vi "Configure Trigger (Timeout).vi"(0 "VISA resource name":refnum<visa-resource-name>, 1 "Timer (500E-12s)":dbl=5e-10, 5 "Source (0:Channel1)":u16(ring) items=["Channel1", "Channel2", "Channel3", "Channel4", "Digital Channel0", "Digital Channel1", "Digital Channel2", "Digital Channel3", "Digital Channel4", "Digital Channel5", "Digital Channel6", "Digital Channel7", "Digital Channel8", "Digital Channel9", "Digital Channel10", "Digital Channel11", "Digital Channel12", "Digital Channel13", "Digital Channel14", "Digital Channel15"], 7 "Trigger Level (0V)":dbl, 9 "Trigger Condition (0:Stays High)":u16(ring) items=["Stays High", "Stays Low", "Either"], 11 "error in (no error)":errorcluster, 12 "Trigger If Timeout (0:Occurs)":u16(ring) items=["Occurs", "Logic"], 13 "Trigger Event (0:A Event)":u16(ring) items=["A Event", "B Event"]) -> (4 "VISA resource name out":refnum<visa-resource-name>, 6 "Trigger Event Out":u16(ring) items=["A Event", "B Event"], 15 "error out":errorcluster)   [LabVIEW 2011, in "Tektronix 7000 Series.lvlib"]
doc: "Configures the timeout trigger settings for an oscilloscope. A timeout occurs when the pulse train stops in the selected state for longer than the specified time.\n\nTDS5000 ,TDS5000B,TDS6000 ,CSA7000 and TDS7000 series oscilloscopes don't support B Timeout Trigger."
uses:
  Tektronix 7000 Series.lvlib
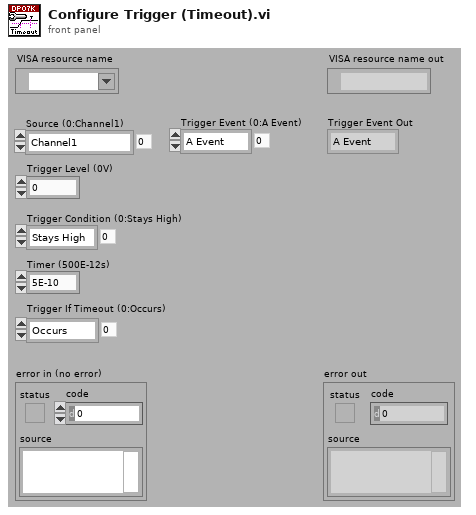
[diagram p1: front panel]
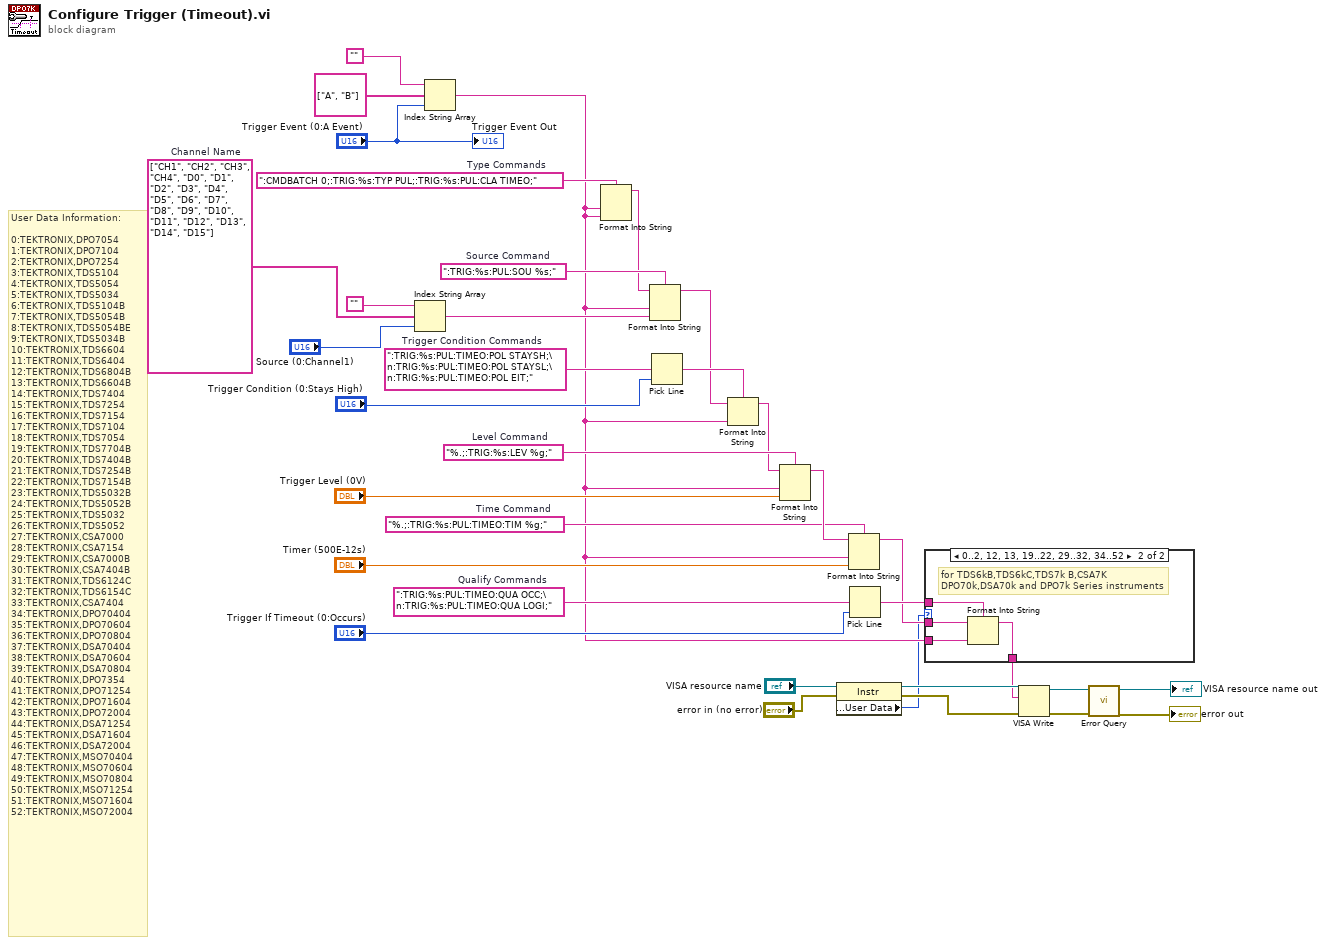
[diagram p0: block diagram]
diagram:
  w1 = string[] ["CH1", "CH2", "CH3", "CH4", "D0", "D1", "D2", "D3", "D4", "D5", "D6", "D7", "D8", "D9", "D10", "D11", "D12", "D13", "D14", "D15"]  # Channel Name
  w21 = "%.;:TRIG:%s:PUL:TIMEO:TIM %g;"  # Time Command
  w23 = "%.;:TRIG:%s:LEV %g;"  # Level Command
  w24 = ":TRIG:%s:PUL:TIMEO:QUA OCC;\n:TRIG:%s:PUL:TIMEO:QUA LOGI;"  # Qualify Commands
  w25 = ":TRIG:%s:PUL:TIMEO:POL STAYSH;\n:TRIG:%s:PUL:TIMEO:POL STAYSL;\n:TRIG:%s:PUL:TIMEO:POL EIT;"  # Trigger Condition Commands
  w26 = ":TRIG:%s:PUL:SOU %s;"  # Source Command
  w20 = ":CMDBATCH 0;:TRIG:%s:TYP PUL;:TRIG:%s:PUL:CLA TIMEO;"  # Type Commands
  # "User Data Information:\n\n0:TEKTRONIX,DPO7054\n1:TEKTRONIX,DPO7104\n2:TEKTRONIX,DPO7254\n3:TEKTRONIX,TDS5104\n4:TEKTRONIX,TDS5054\n5:TEKTRONIX,TDS5034\n6:TEKTRONIX,TDS5104B\n7:TEKTRONIX,TDS5054B\n8:TEKTRONIX,TDS5054BE\n9:TEKTRONIX,TDS5034B\n10:TEKTRONIX,TDS6604\n11:TEKTRONIX,TDS6404\n12:TEKTRONIX,TDS6804B\n13:TEKTRONIX,TDS6604B\n14:TEKTRONIX,TDS7404\n15:TEKTRONIX,TDS7254\n16:TEKTRONIX,TDS7154\n17:TEKTRONIX,TDS7104\n18:TEKTRONIX,TDS7054\n19:TEKTRONIX,TDS7704B\n20:TEKTRONIX,TDS7404B\n21:TEKTRONIX,TDS7254B\n22:TEKTRONIX,TDS7154B\n23:TEKTRONIX,TDS5032B\n24:TEKTRONIX,TDS5052B\n25:TEKTRONIX,TDS5032\n26:TEKTRONIX,TDS5052\n27:TEKTRONIX,CSA7000\n28:TEKTRONIX,CSA7154\n29:TEKTRONIX,CSA7000B\n30:TEKTRONIX,CSA7404B\n31:TEKTRONIX,TDS6124C\n32:TEKTRONIX,TDS6154C\n33:TEKTRONIX,CSA7404\n34:TEKTRONIX,DPO70404\n35:TEKTRONIX,DPO70604\n36:TEKTRONIX,DPO70804\n37:TEKTRONIX,DSA70404\n38:TEKTRONIX,DSA70604\n39:TEKTRONIX,DSA70804\n40:TEKTRONIX,DPO7354\n41:TEKTRONIX,DPO71254\n42:TEKTRONIX,DPO71604\n43:TEKTRONIX,DPO72004\n44:TEKTRONIX,DSA71254\n45:TEKTRONIX,DSA71604\n46:TEKTRONIX,DSA72004\n47:TEKTRONIX,MSO70404\n48:TEKTRONIX,MSO70604\n49:TEKTRONIX,MSO70804\n50:TEKTRONIX,MSO71254\n51:TEKTRONIX,MSO71604\n52:TEKTRONIX,MSO72004"
  n1 = Index String Array(1:"Source (0:Channel1)", 2:w1, 3:"") -> (0:w18:string)
  n2 = Index String Array(1:"Trigger Event (0:A Event)", 2:string[] ["A", "B"], 3:"" ("Empty String Constant")) -> (0:w10:string)
  n3 = Format Into String(format string=w20, w10, w10) -> (resulting string=w19:string)  [unwired: 2 in, 1 out]
  n4 = Format Into String(format string=w26, initial string=w19, w10, w18) -> (resulting string=w16:string)  [unwired: 1 in, 1 out]
  n5 = Pick Line(multi-line string=w25, line index="Trigger Condition (0:Stays High)") -> (output string=w17:string)  [unwired: 1 in]
  n6 = Format Into String(format string=w17, initial string=w16, w10) -> (resulting string=w15:string)  [unwired: 1 in, 1 out]
  n7 = Format Into String(format string=w23, initial string=w15, w10, "Trigger Level (0V)") -> (resulting string=w22:string)  [unwired: 1 in, 1 out]
  n8 = property class="Instr"(reference="VISA resource name", error in="error in (no error)") -> (reference out=w7:refnum<visa-resource-name>, error out=w6:errorcluster, "General Settings:User Data"=w5:u32)
  n9 = Format Into String(format string=w21, initial string=w22, w10, "Timer (500E-12s)") -> (resulting string=w11:string)  [unwired: 1 in, 1 out]
  n10 = Pick Line(multi-line string=w24, line index="Trigger If Timeout (0:Occurs)") -> (output string=w12:string)  [unwired: 1 in]
  n11 = case shown="0..2, 12, 13, 19..22, 29..32, 34..52" w5 {
    tunnel: w12 -> [_ w40]
    tunnel: w11 -> [w36 w39]
    tunnel: w10 -> [_ w38]
    tunnel: [w36 w37] -> w4
    frame Default {
    }
    frame 0..2, 12, 13, 19..22, 29..32, 34..52 {
      # "for TDS6kB,TDS6kC,TDS7k B,CSA7K\nDPO70k,DSA70k and DPO7k Series instruments"
      n12 = Format Into String(format string=w40, initial string=w39, w38) -> (resulting string=w37:string)  [unwired: 1 in, 1 out]
    }
  }
  n13 = VISA Write(VISA resource name=w7, write buffer=w4, error in (no error)=w6) -> (VISA resource name out=w32:refnum<visa-resource-name>, error out=w31:errorcluster)  [unwired: 1 out]
  n14 = call "Error Query.vi"("error in (no error)"=w31, "VISA resource name"=w32) -> ("error out"=→"error out":errorcluster, "VISA resource name out"=→"VISA resource name out":refnum<visa-resource-name>)  [unwired: 6 in, 2 out]
  "Trigger Event Out" <- "Trigger Event (0:A Event)"
